vi "GetActualGFOutput.vi"(0 "Number":T2 items=["1", "2"], 5 "error in":T1) -> (14 "Value":sgl format="%#_g V", 19 "error out":T1)   [LabVIEW 2016]
doc: "Returns the current general transfer function output. The \"number\" identifies the transfer function (0 or 1)."
uses:
  Controls/Generic-Feedback-Number_Selection.ctl
  Controls/Error_Out.ctl
  Files_ASC500/DLL/ASC500_RemoteControlV27.dll
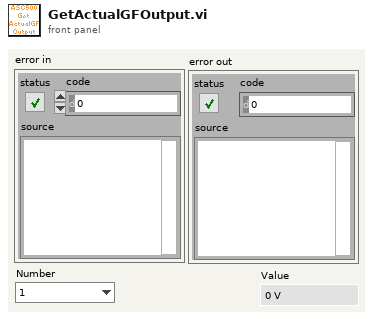
[diagram p1: front panel]
types:
  T1 = typedef "Error_Out.ctl" = errorcluster
  T2 = typedef "Generic-Feedback-Number_Selection.ctl" = i32
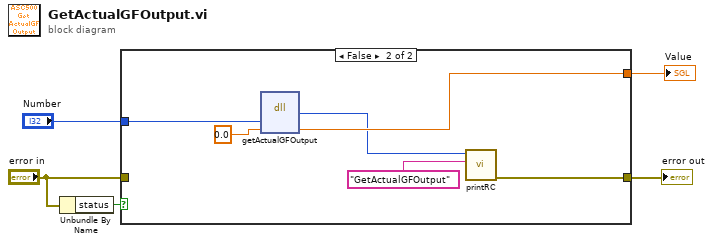
[diagram p0: block diagram]
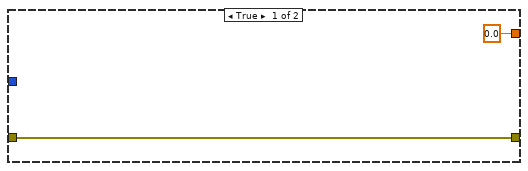
[diagram p2: hidden frame]
diagram:
  n1 = Unbundle By Name("error in") -> ("status"=w5:bool)
  n2 = case shown="False" w5 {
    tunnel: "Number" -> [_ w12]
    tunnel: [sgl 0.0 ("Value") w11] -> w3
    tunnel: [w6 w8] -> w2
    tunnel: "error in" -> [w6 _]
    frame True {
    }
    frame False {
      n3 = dll-call lib="G:/SCMOperations/Share/ELE/Produkt Information/ASC500/04 Remote Control/02 development versions/2018Nov06/Files_ASC500/DLL/ASC500_RemoteControlV27.dll" fn="getActualGFOutput"("Number"=w12, "Value"=sgl 0.0) -> ("return type"=w10:i32, "Value"=w11:sgl)  [unwired: 4 in, 2 out]
      n4 = call "printRC.vi"("additional information"="GetActualGFOutput", "RC"=w10) -> ("error out"=w8:T1)  [unwired: 9 in]
    }
  }
  "error out" <- w2
  "Value" <- w3
